vi "Read Steering Frame.vi"(8 "error in (no error)":errorcluster, 11 "ROV in":refnum<class "ROV Host.lvclass">) -> (0 "error out":errorcluster, 3 "ROV out":refnum<class "ROV Host.lvclass">, 4 "Teleop command":T1)   [LabVIEW 2012, in "ROV Host.lvclass"]
doc: "This VI is used to generate the specific motor commands within the Teleop command message by extracting the angular velocities from each wheel within both frames.\nRuffin"
uses:
  ROV Host.lvclass
  Teleop command.ctl
  ROV Host.lvclass/ROV Host.ctl
  <vilib>/robotics/Steering/Steering Frame/NI_Robotics_Steering Frame.lvclass/NI_Robotics_Steering Frame.ctl
  Support/Host globals (robot acquires video).vi
  <vilib>/robotics/Steering/Steering Frame/NI_Robotics_Steering Frame.lvclass
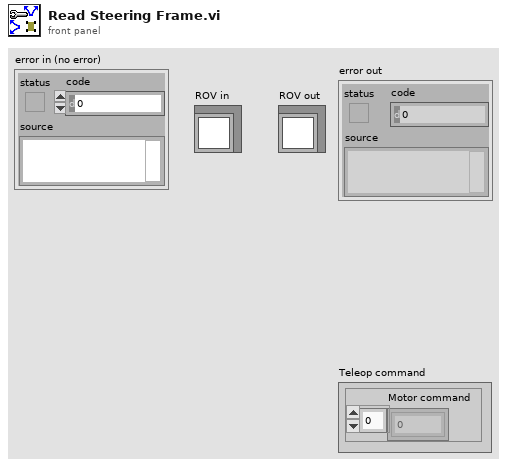
[diagram p1: front panel]
types:
  T1 = typedef "ROV Host.lvclass/Teleop command.ctl" = cluster{"Motor command":i8[]}
  T2 = typedef "NI_Robotics_Steering Class Types.lvlib/Mecanum Steering Frame.ctl" = refnum<class "NI_Robotics_Mecanum Steering Frame.lvclass">
  T3 = typedef "NI_Robotics_Steering Class Types.lvlib/Differential Steering Frame.ctl" = refnum<class "NI_Robotics_Differential Steering Frame.lvclass">
  T4 = typedef "NI_Robotics_Wheel.lvclass/Wheel State.ctl" = cluster{"wheel name":string, "forward angular velocity":dbl, "caster angular velocity":dbl, "caster wheel angle (rad)":dbl, "steering angle (rad)":dbl}
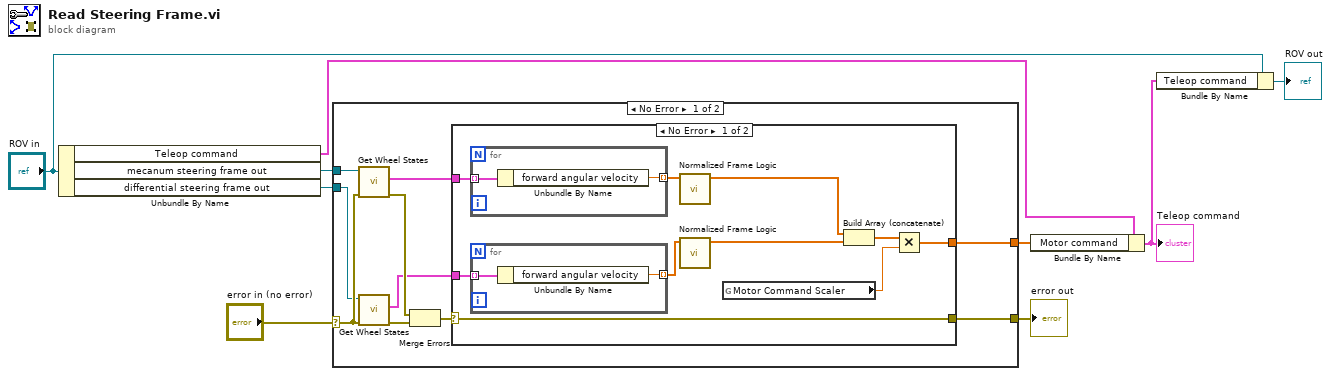
[diagram p0: block diagram]
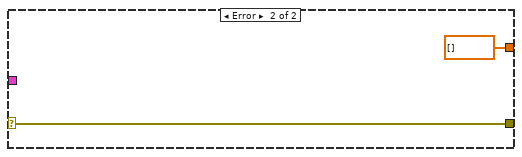
[diagram p2: hidden frame]
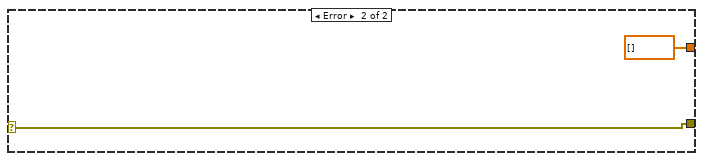
[diagram p3: hidden frame]
diagram:
  n1 = Unbundle By Name("ROV in") -> ("Teleop command"=w4:cluster{"Motor command":dbl[]}, "mecanum steering frame out"=w6:T2, "differential steering frame out"=w5:T3)
  n2 = case shown="No Error" "error in (no error)" {
    selector: "error in (no error)" -> [w12 w37]
    tunnel: [w15 w37] -> w7
    tunnel: w6 -> [w14 _]
    tunnel: w5 -> [w11 _]
    tunnel: [w13 dbl[] []] -> w3
    frame No Error {
      n3 = call <vilib>:"Get Wheel States.vi"("error in (no error)"=w12, "steering frame in"=w14) -> ("error out"=w18:errorcluster, "wheel states"=w16:T4[])  [unwired: 7 in, 1 out]
      n4 = call <vilib>:"Get Wheel States.vi"("error in (no error)"=w12, "steering frame in"=w11) -> ("error out"=w19:errorcluster, "wheel states"=w10:T4[])  [unwired: 7 in, 1 out]
      n5 = Merge Errors(w18, w19) -> (w17:errorcluster)
      n6 = case shown="No Error" w17 {
        selector: w17 -> [w29 w35]
        tunnel: w16 -> [w28 _]
        tunnel: w10 -> [w27 _]
        tunnel: [w29 w35] -> w15
        tunnel: [w25 dbl[] []] -> w13
        frame No Error {
          n7 = for {
            tunnel: w28 -> [w32] mode=indexing
            tunnel: [w33] -> w24 mode=indexing
            n8 = Unbundle By Name(w32) -> ("forward angular velocity"=w33:dbl)
          }
          n9 = for {
            tunnel: w27 -> [w30] mode=indexing
            tunnel: [w31] -> w23 mode=indexing
            n10 = Unbundle By Name(w30) -> ("forward angular velocity"=w31:dbl)
          }
          n11 = call "Normalized Frame Logic.vi"("Array in"=w24) -> ("Array out"=w21:dbl[])  [unwired: 10 in]
          n12 = call "Normalized Frame Logic.vi"("Array in"=w23) -> ("Array out"=w22:dbl[])  [unwired: 10 in]
          n13 = global read "Host globals (robot acquires video).vi" "Motor Command Scaler"() -> (w20:dbl)
          n14 = Build Array (concatenate)(w21, w22) -> (w26:dbl[])
          n15 = Multiply(x=w26, y=w20) -> (x*y=w25:dbl[])
        }
        frame Error {
        }
      }
    }
    frame Error {
    }
  }
  "error out" <- w7
  n16 = Bundle By Name(cluster=w4, "Motor command"=w3) -> (w1:cluster{"Motor command":dbl[]})
  "Teleop command" <- w1
  n17 = Bundle By Name(cluster="ROV in", "Teleop command"=w1) -> (→"ROV out":refnum<class "ROV Host.lvclass">)
